vi "Change file name extension.vi"(3 "New Extension (no period)":string="html", 4 "Path String In":string) -> (0 "New Path String Out":string, 1 "New Path Out":path)   [LabVIEW 2015]
doc: "Changes the extension of a filename (i.e., the characters following the last period in the name) to the specified string. The period and extension are simply appended to the name if they are not already there."
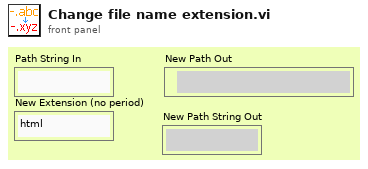
[diagram p1: front panel]
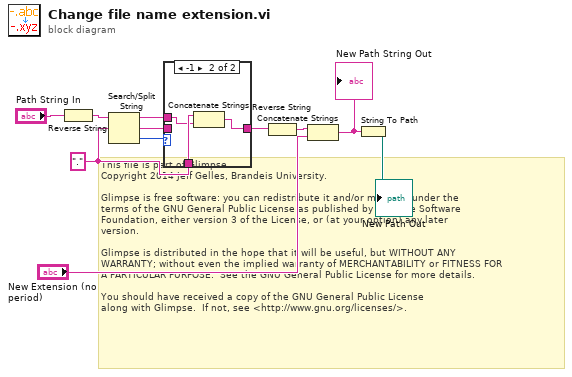
[diagram p0: block diagram]
diagram:
  w2 = "." ("search string/char (-)")
  # "This file is part of Glimpse. \nCopyright 2014 Jeff Gelles, Brandeis University.    \n\nGlimpse is free software: you can redistribute it and/or modify it under the \nterms of the GNU General Public License as published by the Free Software \nFoundation, either version 3 of the License, or (at your option) any later \nversion.\n\nGlimpse is distributed in the hope that it will be useful, but WITHOUT ANY \nWARRANTY; without even the implied warranty of MERCHANTABILITY or FITNESS FOR \nA PARTICULAR PURPOSE.  See the GNU General Public License for more details.\n\nYou should have received a copy of the GNU General Public License\nalong with Glimpse.  If not, see <http://www.gnu.org/licenses/>."
  n1 = Reverse String(1:"Path String In") -> (0:w7:string)
  n2 = Search/Split String(string=w7, search string/char (-)=w2) -> (substring before match=w1:string, match + rest of string=w4:string, offset of match=w5:i32)  [unwired: 1 out]
  n3 = case shown="-1" w5 {
    tunnel: w4 -> [w12 _]
    tunnel: [w12 w13] -> w3
    tunnel: w2 -> [_ w15]
    tunnel: w1 -> [_ w14]
    frame 0, Default {
    }
    frame -1 {
      n4 = Concatenate Strings(w15, w14) -> (w13:string)
    }
  }
  n5 = Reverse String(1:w3) -> (0:w8:string)
  n6 = Concatenate Strings(w8, "New Extension (no period)") -> (w10:string)
  "New Path String Out" <- w10
  n7 = String To Path(string=w10) -> (path=→"New Path Out":path)
